vi "Initialize - Section Page Panel.vi"(7 "Packets Listbox":refnum<vi>, 8 "error in (no error)":errorcluster, 11 "Item Ref in":T1 format="%.0x") -> (0 "error out":errorcluster, 3 "Item Ref out":T1 format="%.0x")   [LabVIEW 2016, in "UDP-Custom-Device System Explorer.lvlib"]
doc: "Initialize the Rx Channels Section Page Panel."
uses:
  UDP-Custom-Device System Explorer.lvlib
  <vilib>/NI Veristand/Custom Device API/Custom Device Item Ref.ctl
  <vilib>/Utility/miscctls.llb/LVRowAndColumnUnsignedTypeDef.ctl
  Property Accessors/Shared Section Accessors.lvlib
  Property Accessors/Shared Packet Accessors.lvlib
  <vilib>/NI VeriStand/Custom Device API/Custom Device API.lvlib
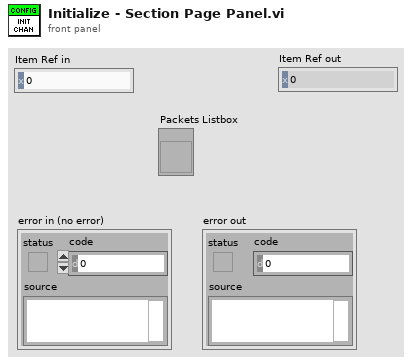
[diagram p1: front panel]
types:
  T1 = typedef "Custom Device API.lvlib/Custom Device Item Ref.ctl" = u64
  T2 = typedef "LVRowAndColumnUnsignedTypeDef.ctl" = cluster{"Row":u32, "Column":u32}
  T3 = typedef "Custom Device API.lvlib/Custom Device Item Info.ctl" = cluster{"Name":string, "Is Channel":bool, "GUID":string, "Is Waveform":bool}
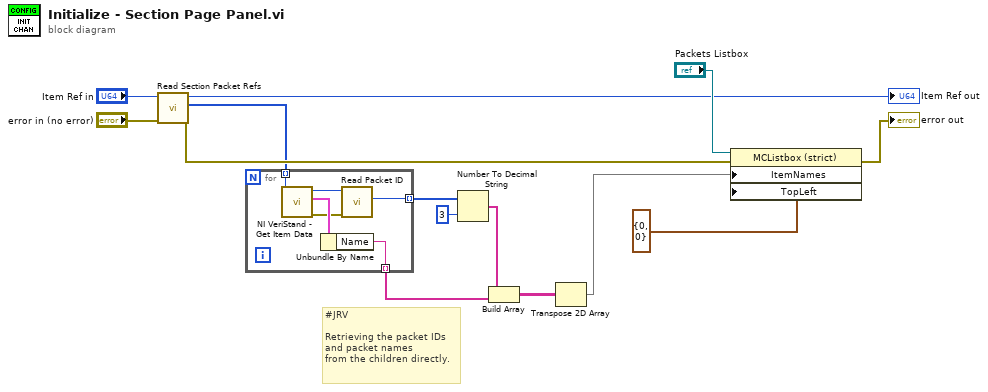
[diagram p0: block diagram]
diagram:
  # "#JRV\n\nRetrieving the packet IDs\nand packet names \nfrom the children directly."
  n1 = call "Read Section Packet Refs.vi"("error in (no error)"="error in (no error)", "Node Ptr"="Item Ref in") -> ("error out"=w2:errorcluster, "Dependent Node Refs"=w1:T1[], "Node Ptr out"=→"Item Ref out":T1)  [unwired: 7 in]
  n2 = for {
    tunnel: w1 -> [w18] mode=indexing
    tunnel: [w20] -> w8 mode=indexing
    tunnel: [w16] -> w7 mode=indexing
    n3 = call <vilib>:"NI VeriStand - Get Item Data.vi"("Item Ref in"=w18) -> ("error out"=w17:errorcluster, "Item Info"=w19:T3, "Item Ref out"=w15:T1)  [unwired: 7 in, 1 out]
    n4 = Unbundle By Name(w19) -> ("Name"=w16:string)
    n5 = call "Read Packet ID.vi"("error in (no error)"=w17, "Node Ptr"=w15) -> ("Packet ID"=w20:i32)  [unwired: 7 in, 2 out]
  }
  n6 = Number To Decimal String(number=w8, width (-)=i16 3) -> (decimal integer string=w9:string[])
  n7 = Build Array(w9, w7) -> (w12:string[][])
  n8 = Transpose 2D Array(2D array=w12) -> (transposed array=w13:string[][])
  n9 = property class="MCListbox (strict)"(reference="Packets Listbox", error in=w2, "ItemNames"=w13, "TopLeft"=T2 {"Row"=0, "Column"=0} ("Top Left Visible Cell")) -> (error out=→"error out":errorcluster)  [unwired: 1 out]
